vi "PPMS.Chamber Action to Ring.vi"(1 "Data in":T1="Seal") -> (0 "Value":u16=1)   [LabVIEW 2019, in "instrument.PPMS.lvclass"]
uses:
  instrument.PPMS.lvclass
  Typedefs/PPMS.Chamber Command--enum.ctl
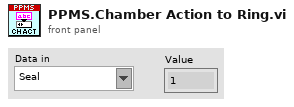
[diagram p1: front panel]
types:
  T1 = typedef "instrument.PPMS.lvclass/PPMS.Chamber Command--enum.ctl" = string
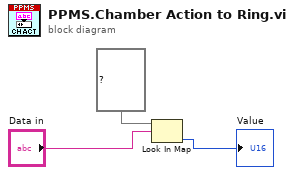
[diagram p0: block diagram]
diagram:
  n1 = Look In Map(map=map{string, u16} {"HighVacuum"=5, "PumpContinuous"=3, "PurgeAndSeal"=1, "Seal"=0, "VentAndSeal"=2, "VentContinuous"=4} ("Map"), key="Data in") -> (value=→"Value":u16)  [unwired: 1 in, 1 out]
